vi "Set DDG Step Coefficients.vi"(9 "p2":dbl, 10 "p1":dbl, 11 "mode":u32) -> (3 "function return":u32)   [LabVIEW 2018, in "AndorSDK.lvlib"]
doc: "EXPNETTYPE unsigned int WINAPI SetDDGStepCoefficients(at_u32 mode, double p1, double p2);"
uses:
  AndorSDK.lvlib
  ATMCD32D.dll
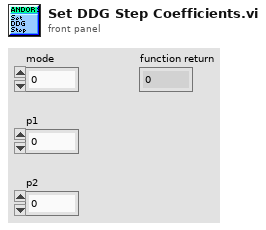
[diagram p1: front panel]
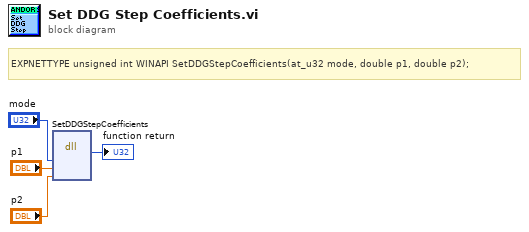
[diagram p0: block diagram]
diagram:
  # "EXPNETTYPE unsigned int WINAPI SetDDGStepCoefficients(at_u32 mode, double p1, double p2);"
  n1 = dll-call lib="PTH2babs E\nPersönliches02 - Arbeit03-HiwijobsLabviewCodelibANDOR\tAndor SDK\nATMCD32D.*" fn="SetDDGStepCoefficients"("mode"="mode", "p1"="p1", "p2"="p2") -> (→"function return":u32)  [unwired: 6 in, 2 out]
